vi "Test.vi"() -> ()   [LabVIEW 2019]
uses:
  LifterSUBVis/Motor Class/Lifter_motor.lvclass
panel:
  out "step out":i32
  out "error out":errorcluster
  in  "New one":bool
  out "AI2":dbl
  out "AI0":dbl
  in  "n_samples 3":i32=10
  out "Execution Time 3":u32
  in  "Boolean":bool
  in  "File Name":string
  out "Execution Time":u32
  out "ADC Voltage":dbl format="%0.2f"
  in  "n_samples":i32=10
  out "Driver ACK?":bool
  in  "Direction":bool
  out "Upper Limmit":bool
  out "Top":bool
  out "Anneal":bool
  out "Middle":bool
  out "Bottom":bool
  out "Home":bool
  out "Lower Limit":bool
  out "Step Count":i32
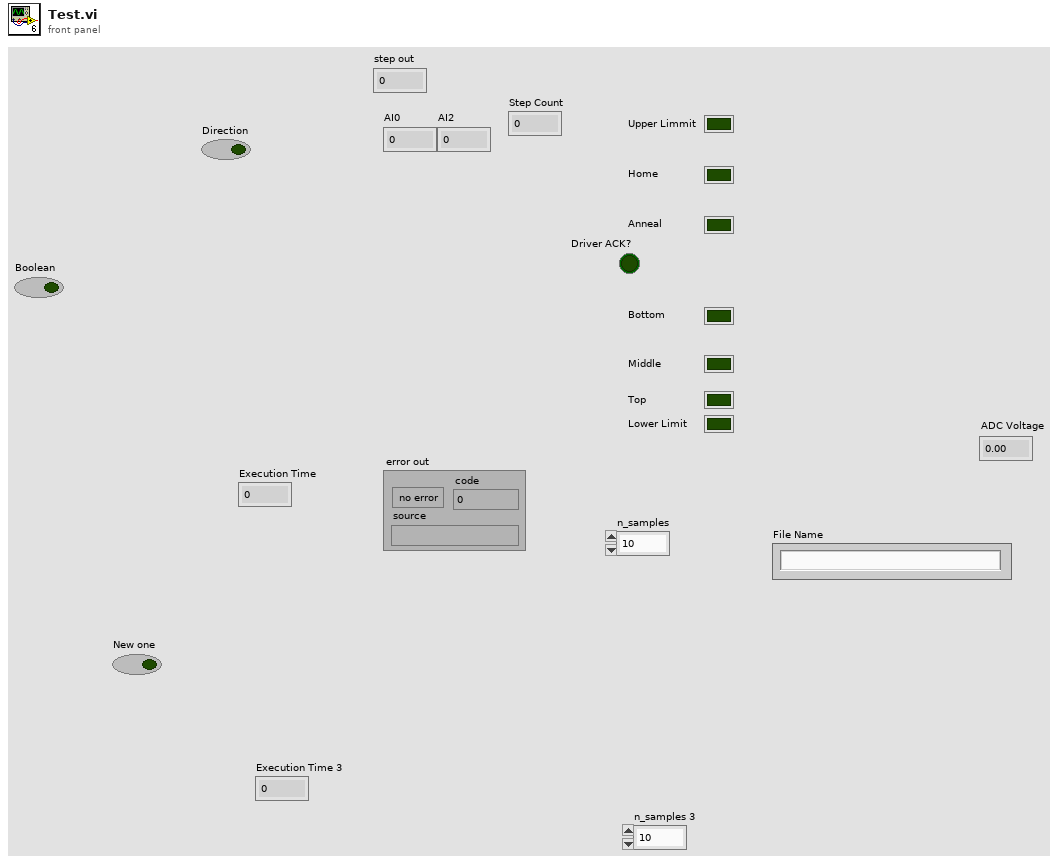
[diagram p1: front panel]
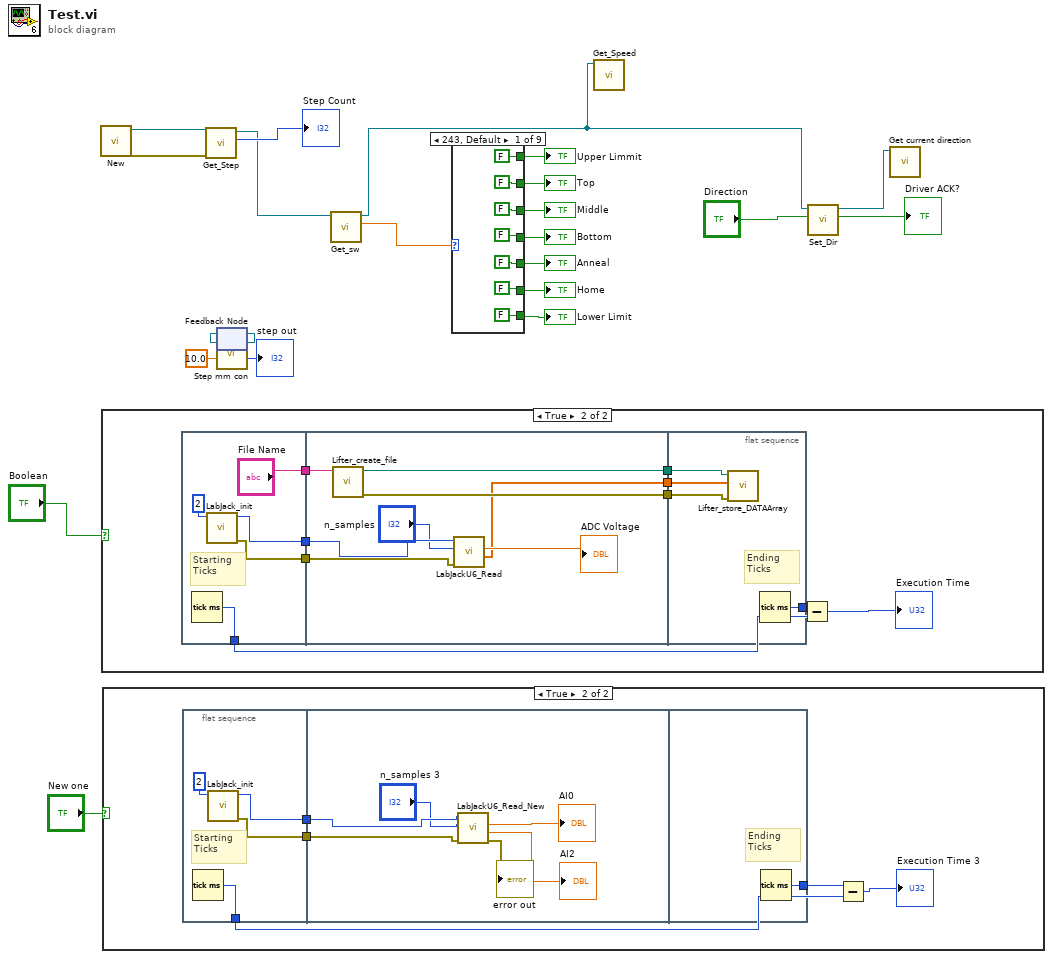
[diagram p0: block diagram]
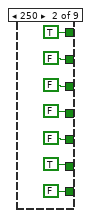
[diagram p4: hidden frame]
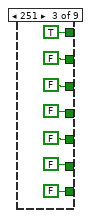
[diagram p5: hidden frame]
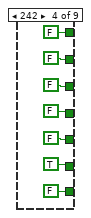
[diagram p6: hidden frame]
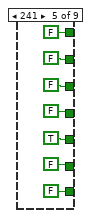
[diagram p7: hidden frame]
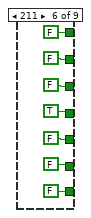
[diagram p8: hidden frame]
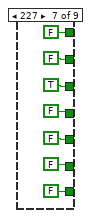
[diagram p9: hidden frame]
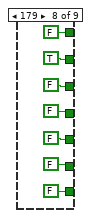
[diagram p10: hidden frame]
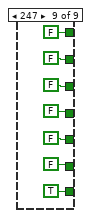
[diagram p11: hidden frame]
diagram:
  n1 = call "New.vi"() -> ("error out"=w22:errorcluster, "Lifter_motor out"=w21:refnum<class "Lifter_motor.lvclass">)  [unwired: 10 in]
  n2 = case shown="True" "Boolean" {
    frame False {
    }
    frame True {
      n3 = flat-sequence {
        tunnel: [w36] -> w24
        tunnel: [w35] -> w31
        tunnel: [w34] -> w30
        tunnel: ["File Name"] -> w29
        tunnel: w31 -> [w43]
        tunnel: w30 -> [w42]
        tunnel: w29 -> [w40]
        tunnel: [w39] -> w28
        tunnel: [w38] -> w27
        tunnel: [w37] -> w26
        tunnel: [w48] -> w25
        tunnel: w28 -> [w46]
        tunnel: w27 -> [w47]
        tunnel: w26 -> [w45]
        frame #0 {
          # "Starting Ticks"
          n4 = Tick Count (ms)() -> (millisecond timer value=w36:u32)
          n5 = call "LabJack_init.vi"("Positive Channel #"=2) -> ("error out"=w35:errorcluster, "Handle Out"=w34:i32)  [unwired: 8 in, 1 out]
        }
        frame #1 {
          n6 = call "Lifter_create_file.vi"("File Name"=w40) -> ("error out"=w38:errorcluster, "dup path"=w39:path)  [unwired: 9 in]
          n7 = call "LabJackU6_Read.vi"("error in"=w43, "n_samples"="n_samples", "Handle In"=w42) -> ("ADC_Array"=w37:dbl[], "Mean ADC Voltage"=→"ADC Voltage":dbl)  [unwired: 5 in, 2 out]
        }
        frame #2 {
          # "Ending Ticks"
          n8 = call "Lifter_store_DATAArray.vi"("error in (no error)"=w47, "1D data"=w45, "file path (dialog if empty)"=w46) -> ()  [unwired: 5 in, 2 out]
          n9 = Tick Count (ms)() -> (millisecond timer value=w48:u32)
        }
      }
      n10 = Subtract(x=w25, y=w24) -> (x-y=→"Execution Time":u32)
    }
  }
  n11 = case shown="True" "New one" {
    frame False {
    }
    frame True {
      n12 = flat-sequence {
        tunnel: [w57] -> w50
        tunnel: [w56] -> w53
        tunnel: [w55] -> w52
        tunnel: w53 -> [w63]
        tunnel: w52 -> [w62]
        tunnel: [w64] -> w51
        frame #0 {
          # "Starting Ticks"
          n13 = Tick Count (ms)() -> (millisecond timer value=w57:u32)
          n14 = call "LabJack_init.vi"("Positive Channel #"=2) -> ("error out"=w56:errorcluster, "Handle Out"=w55:i32)  [unwired: 8 in, 1 out]
        }
        frame #1 {
          n15 = call "LabJackU6_Read_New.vi"("error in"=w63, "n_samples"="n_samples 3", "Handle In"=w62) -> ("error out"=→"error out":errorcluster, "AI2"=→"AI2":dbl, "AI0"=→"AI0":dbl)  [unwired: 5 in, 1 out]
        }
        frame #2 {
          # "Ending Ticks"
          n16 = Tick Count (ms)() -> (millisecond timer value=w64:u32)
        }
      }
      n17 = Subtract(x=w51, y=w50) -> (x-y=→"Execution Time 3":u32)
    }
  }
  n18 = call "Get_Step.vi"("error in (no error)"=w22, "Lifter_motor in"=w21) -> ("Step Count"=→"Step Count":i32, "Lifter_motor out"=w12:refnum<class "Lifter_motor.lvclass">)  [unwired: 7 in, 1 out]
  n19 = feedback #1() -> (w3:refnum<class "Lifter_motor.lvclass">)  [unwired: 1 in]
  n20 = call "Step mm con.vi"("mm in"=10.0, "Lifter_motor in"=w3) -> ("step out"=→"step out":i32, "Lifter_motor out"=w4:refnum<class "Lifter_motor.lvclass">)  [unwired: 6 in, 2 out]
  n21 = feedback-in #1(w4) -> ()
  n22 = call-dynamic "Get_sw.vi"("Lifter_motor in"=w12) -> ("Switch Hex"=w11:dbl, "Lifter_motor out"=w8:refnum<class "Lifter_motor.lvclass">)  [unwired: 8 in, 1 out]
  n23 = case shown="243, Default" w11 {
    tunnel: [FALSE ("Lower Limit") TRUE ("Lower Limit") TRUE ("Lower Limit") FALSE ("Lower Limit") FALSE ("Lower Limit") FALSE ("Lower Limit") FALSE ("Lower Limit") FALSE ("Lower Limit") FALSE ("Lower Limit")] -> w19
    tunnel: [FALSE ("Lower Limit") FALSE ("Lower Limit") FALSE ("Lower Limit") FALSE ("Lower Limit") FALSE ("Lower Limit") FALSE ("Lower Limit") FALSE ("Lower Limit") TRUE ("Lower Limit") FALSE ("Lower Limit")] -> w18
    tunnel: [FALSE ("Lower Limit") FALSE ("Lower Limit") FALSE ("Lower Limit") FALSE ("Lower Limit") FALSE ("Lower Limit") FALSE ("Lower Limit") TRUE ("Lower Limit") FALSE ("Lower Limit") FALSE ("Lower Limit")] -> w17
    tunnel: [FALSE ("Lower Limit") FALSE ("Lower Limit") FALSE ("Lower Limit") FALSE ("Lower Limit") FALSE ("Lower Limit") TRUE ("Lower Limit") FALSE ("Lower Limit") FALSE ("Lower Limit") FALSE ("Lower Limit")] -> w16
    tunnel: [FALSE ("Lower Limit") FALSE ("Lower Limit") FALSE ("Lower Limit") FALSE ("Lower Limit") TRUE ("Lower Limit") FALSE ("Lower Limit") FALSE ("Lower Limit") FALSE ("Lower Limit") FALSE ("Lower Limit")] -> w15
    tunnel: [FALSE ("Lower Limit") TRUE ("Lower Limit") FALSE ("Lower Limit") TRUE ("Lower Limit") FALSE ("Lower Limit") FALSE ("Lower Limit") FALSE ("Lower Limit") FALSE ("Lower Limit") FALSE ("Lower Limit")] -> w14
    tunnel: [FALSE ("Lower Limit") FALSE ("Lower Limit") FALSE ("Lower Limit") FALSE ("Lower Limit") FALSE ("Lower Limit") FALSE ("Lower Limit") FALSE ("Lower Limit") FALSE ("Lower Limit") TRUE ("Lower Limit")] -> w13
    frame 243, Default {
    }
    frame 250 {
    }
    frame 251 {
    }
    frame 242 {
    }
    frame 241 {
    }
    frame 211 {
    }
    frame 227 {
    }
    frame 179 {
    }
    frame 247 {
    }
  }
  "Lower Limit" <- w13
  "Home" <- w14
  "Bottom" <- w16
  "Middle" <- w17
  "Anneal" <- w15
  "Top" <- w18
  "Upper Limmit" <- w19
  n24 = call "Get_Speed.vi"("Lifter_motor in"=w8) -> ()  [unwired: 7 in, 4 out]
  n25 = call "Set_Dir.vi"("Direction"="Direction", "Lifter_motor in"=w8) -> ("Driver ACK?"=→"Driver ACK?":bool, "Lifter_motor out"=w5:refnum<class "Lifter_motor.lvclass">)  [unwired: 7 in, 1 out]
  n26 = call "Get current direction.vi"("Lifter_motor in"=w5) -> ()  [unwired: 8 in, 3 out]
